vi "Load APU Setup File.vi"(8 "error in (no error)":errorcluster, 11 "APU Select":T1="<Select>") -> (0 "error out":errorcluster)   [LabVIEW 2018, in "File IO.lvlib"]
doc: "This subVI enqueues the named action in to the communications queue along with the input data."
uses:
  File IO.lvlib
  Controller (Host)/Public Controls/APU Select.ctl
  Private Controls/Module Data.ctl
  Private Controls/Module Action.ctl
  Controller (Host)/Controller (Host).lvlib
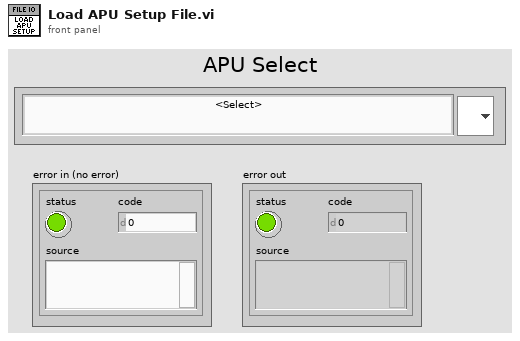
[diagram p1: front panel]
types:
  T1 = typedef "Controller (Host).lvlib/APU Select.ctl" = string
  T2 = typedef "File IO.lvlib/Module Data.ctl" = cluster{"Data":variant, "Action":T3}
  T3 = typedef "File IO.lvlib/Module Action.ctl" = enum8{"Timeout", "OpenReport", "Continue Test", "Init", "Error", "Exit", "Save Accel Data", "Set Recording State", "Log APU RunTime", "Start New Test", "Create New Reports", "Write to System Log", "Save Variables", "Load APU Setup File", "Increment Run Count", "Write To Report"}
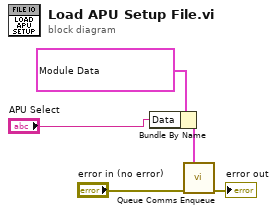
[diagram p0: block diagram]
diagram:
  n1 = Bundle By Name(cluster=T2 {"Data"=variant, "Action"=enum."Load APU Setup File"} ("element"), "Data"="APU Select") -> (w2:T2)
  n2 = call "Queue Comms Enqueue.vi"("error in (no error)"="error in (no error)", "element"=w2) -> ("error out"=→"error out":errorcluster)  [unwired: 9 in]
